vi "Get Components Target Directory.vi"(8 "error in (no error)":errorcluster, 11 "Item Ref in":T1 format="%.0x") -> (0 "error out":errorcluster, 2 "components target directory":path, 3 "Item Ref out":T1 format="%.0x")   [LabVIEW 2020, in "DSF Shared.lvlib"]
uses:
  DSF Shared.lvlib
  <vilib>/NI VeriStand/Custom Device API/Custom Device Item Ref.ctl
  <vilib>/NI VeriStand/Custom Device API/Get Item Property (Path).vi
  <vilib>/NI VeriStand/Custom Device API/Custom Device API.lvlib
  DSF System Explorer.lvlib
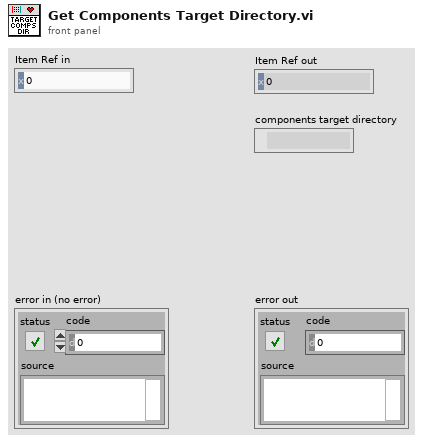
[diagram p1: front panel]
types:
  T1 = typedef "Custom Device API.lvlib/Custom Device Item Ref.ctl" = u64
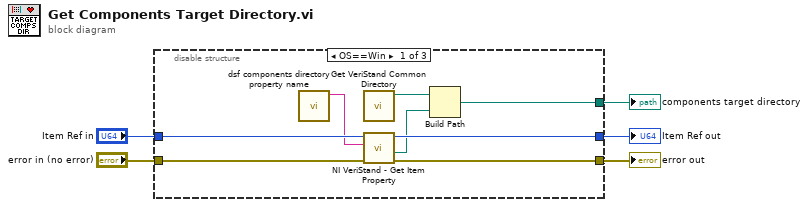
[diagram p0: block diagram]
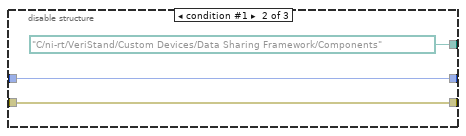
[diagram p2: hidden frame]
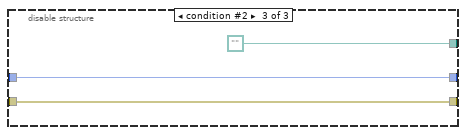
[diagram p3: hidden frame]
diagram:
  n1 = disable-structure shown="OS==Win" {
    disable-tunnel: "Item Ref in" -> [w13 w15 w19]
    disable-tunnel: "error in (no error)" -> [w12 w14 w18]
    disable-tunnel: [w11 w15 w19] -> w2
    disable-tunnel: [w10 w14 w18] -> w3
    disable-tunnel: [w6 path "C:/ni-rt/VeriStand/Custom Devices/Data Sharing Framework/Components" ("RT Destination") path "" ("appended path")] -> w1
    frame condition #0 (active) {
      n2 = call "dsf components directory property name.vi"() -> ("components directory property name"=w9:string)  [unwired: 11 in]
      n3 = call "Get VeriStand Common Directory.vi"() -> ("common directory"=w8:path)  [unwired: 11 in]
      n4 = call-poly <vilib>:"NI VeriStand - Get Item Property.vi"("error in (no error)"=w12, "Property Name"=w9, "Item Ref in"=w13) -> ("error out"=w10:errorcluster, "Value"=w7:path, "Item Ref out"=w11:T1)  [unwired: 5 in, 1 out]
      n5 = Build Path(base path=w8, name or relative path=w7) -> (appended path=w6:path)
    }
    frame condition #1 {
    }
    frame condition #2 {
    }
  }
  "Item Ref out" <- w2
  "error out" <- w3
  "components target directory" <- w1
